vi "MGCC_StaEst_pnjoc.vi"(0 "MeaPha":T2, 1 "Num":T1, 2 "StateVar":dbl[](array[numeric]), 3 "B":dbl[][](array[numeric]), 4 "G":dbl[][](array[numeric])) -> (5 "joc_pn":dbl[][](array[numeric]), 6 "joc_qn":dbl[][](array[numeric]))   [LabVIEW 2016]
uses:
  <vilib>/imath/engines/lvmath2/RunTimeEngine/RunTimeType/NIMS_RunTimeType_From StrictType (excl LVString).vi
  <instcachedir>/0/NIMS_RunTimeType_From StrictType (excl LVString)_BBF44FB49F834B71AF7A14CCEDF8BECD.lvgen/NIMS_RunTimeType_From StrictType (excl LVString)_BBF44FB49F834B71AF7A14CCEDF8BECD_032.vi
  <instcachedir>/0/NIMS_RunTimeType_From StrictType (excl LVString)_BBF44FB49F834B71AF7A14CCEDF8BECD.lvgen/NIMS_RunTimeType_From StrictType (excl LVString)_BBF44FB49F834B71AF7A14CCEDF8BECD_031.vi
  <vilib>/imath/engines/lvmath2/RunTimeEngine/Struct/NIMS_StructSetField.vi
  <instcachedir>/0/NIMS_RunTimeType_From StrictType (excl LVString)_BBF44FB49F834B71AF7A14CCEDF8BECD.lvgen/NIMS_RunTimeType_From StrictType (excl LVString)_BBF44FB49F834B71AF7A14CCEDF8BECD_024.vi
  <vilib>/imath/engines/lvmath2/RunTimeEngine/Struct/NIMS_StructGetField.vi
  <vilib>/imath/engines/lvmath2/RunTimeEngine/RunTimeType/NIMS_RunTimeType_To Numeric.vi
  <instcachedir>/0/NIMS_RunTimeType_To Numeric_19D51BCABB82435A94073491761E42EE.lvgen/NIMS_RunTimeType_To Numeric_19D51BCABB82435A94073491761E42EE_010.vi
  <vilib>/imath/engines/lvmath2/RunTimeEngine/BuiltInFunctions/size/NIMS_I32=size(GM,I32).vi
  <instcachedir>/0/NIMS_I32=size(GM,I32)_122058B1B3294FAEA5DC209B92B394E4.lvgen/NIMS_I32=size(GM,I32)_122058B1B3294FAEA5DC209B92B394E4_005.vi
  <vilib>/imathl/engines/lvmath/Functions/Error Handling/Create Error.vi
  <instcachedir>/0/NIMS_RunTimeType_To Numeric_19D51BCABB82435A94073491761E42EE.lvgen/NIMS_RunTimeType_To Numeric_19D51BCABB82435A94073491761E42EE_008.vi
  <instcachedir>/0/NIMS_RunTimeType_To Numeric_19D51BCABB82435A94073491761E42EE.lvgen/NIMS_RunTimeType_To Numeric_19D51BCABB82435A94073491761E42EE_009.vi
  <vilib>/imath/engines/lvmath2/RunTimeEngine/BuiltInFunctions/zeros/NIMS_M=zeros(I32,I32).vi
  <vilib>/imath/engines/lvmath2/RunTimeEngine/BuiltInFunctions/zeros/NIMS_V=zeros(I32,I32).vi
  <vilib>/imath/engines/lvmath2/RunTimeEngine/RangeToken/NIMS_Range_R2 - Integer.vi
  <instcachedir>/0/NIMS_Range_R2 - Integer_89B873E74E6E489885E44F751DD9C6BF.lvgen/NIMS_Range_R2 - Integer_89B873E74E6E489885E44F751DD9C6BF_000.vi
  <vilib>/imath/engines/lvmath2/RunTimeEngine/CommandStatement/MC_CommandStatement_break.vi
  <vilib>/imath/engines/lvmath2/RunTimeEngine/IndexRead/NIMS M(S,S).vi
  <instcachedir>/0/NIMS M(S,S)_AC51E74150A542F7991B9634C66F3096.lvgen/NIMS M(S,S)_AC51E74150A542F7991B9634C66F3096_002.vi
  <vilib>/imath/engines/lvmath2/RunTimeEngine/RangeToken/NIMS_Range_R2 - Float.vi
  <instcachedir>/0/NIMS_Range_R2 - Float_590A1087448447AEB7F770FC082D3801.lvgen/NIMS_Range_R2 - Float_590A1087448447AEB7F770FC082D3801_000.vi
  <vilib>/imath/engines/lvmath2/RunTimeSupport/NIMS_Error if Not Equal.vi
  <instcachedir>/0/NIMS_Error if Not Equal_43252A79AD05436189442EC0C5E5AB8A.lvgen/NIMS_Error if Not Equal_43252A79AD05436189442EC0C5E5AB8A_000.vi
  <vilib>/imath/engines/lvmath2/RunTimeEngine/IndexRead/NIMS V(S).vi
  <instcachedir>/0/NIMS V(S)_0488751826AF41519A22953C041130DC.lvgen/NIMS V(S)_0488751826AF41519A22953C041130DC_000.vi
  <vilib>/imath/engines/lvmath2/RunTimeEngine/ErrorHandling/NIMS_Create Error From Enums.vi
  <instcachedir>/0/NIMS M(S,S)_AC51E74150A542F7991B9634C66F3096.lvgen/NIMS M(S,S)_AC51E74150A542F7991B9634C66F3096_000.vi
  <vilib>/imath/engines/lvmath2/RunTimeEngine/IndexReplace/NIMS M(S,S)=S.vi
  <instcachedir>/0/NIMS M(S,S)=S_98E40400474E4398B113AE20298B4F82.lvgen/NIMS M(S,S)=S_98E40400474E4398B113AE20298B4F82_000.vi
  <vilib>/imath/engines/lvmath2/RunTimeEngine/IndexReplace/NIMS V(S)=S.vi
  <instcachedir>/0/NIMS V(S)=S_57E16554CB8B4B90AAB163894F717546.lvgen/NIMS V(S)=S_57E16554CB8B4B90AAB163894F717546_000.vi
  <vilib>/imath/engines/lvmath2/RunTimeEngine/NodeEndStatement/NIMS_NodeEndStatement_Output.vi
  <instcachedir>/0/NIMS_NodeEndStatement_Output_53EC0D466D134D7ABD903AC30B43404B.lvgen/NIMS_NodeEndStatement_Output_53EC0D466D134D7ABD903AC30B43404B_002.vi
  <vilib>/imath/engines/lvmath2/RunTimeEngine/ErrorHandling/NIMS_Finalize Error.vi
panel:
  out "error out":errorcluster
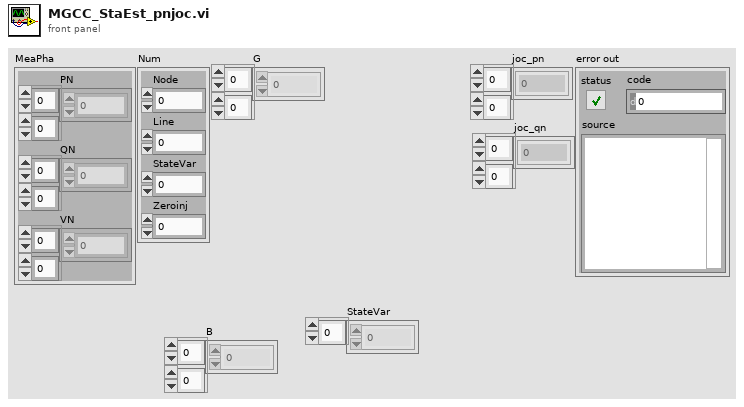
[diagram p1: front panel]
types:
  T1 = cluster{"Node":dbl, "Line":dbl, "StateVar":i32, "Zeroinj":i32}
  T2 = cluster{"PN":i32[][], "QN":i32[][], "VN":i32[][]}
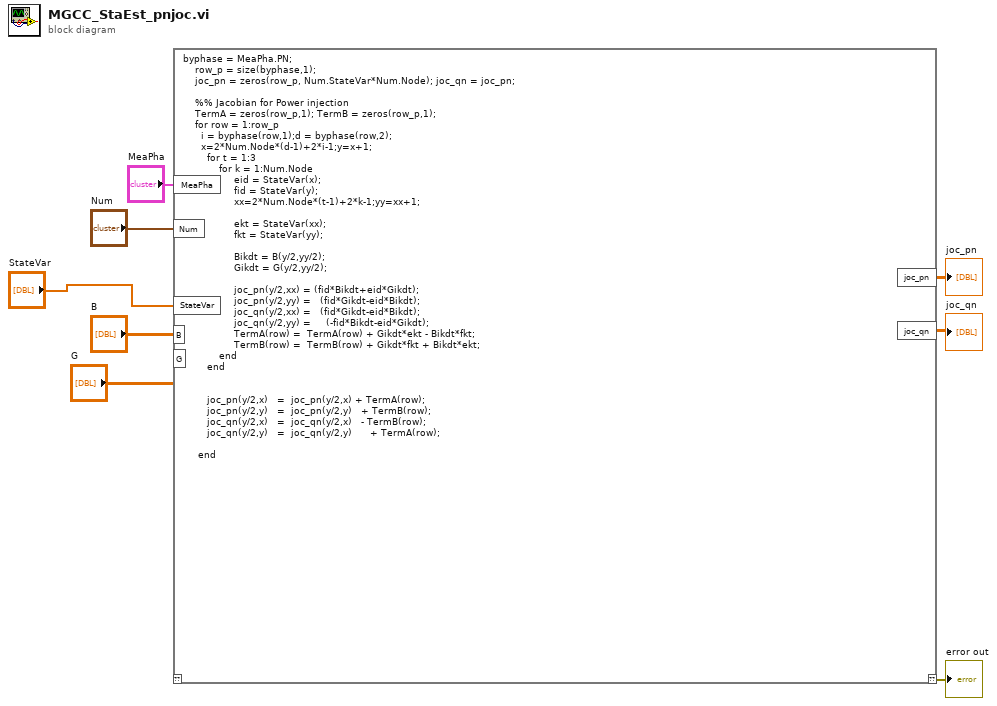
[diagram p0: block diagram]
diagram:
  n1 = mathscript code="byphase = MeaPha.PN;    \n    row_p = size(byphase,1);\n    joc_pn = zeros(row_p, Num.StateVar*Num.Node); joc_qn = joc_pn;\n    \n    %% Jacobian for Power injection\n    TermA = zeros(row_p,1); TermB = zeros(row_p,1);\n    for row = 1:row_p\n      i = byphase(row,1);d = byphase(row,2);\n      x=2*Num.Node*(d-1)+2*i-1;y=x+1;\n        for t = 1:3\n            for k = 1:Num.Node \n                 eid = StateVar(x);\n                 fid = StateVar(y);\n                 xx=2*Num.Node*(t-1)+2*k-1;yy=xx+1;\n\n                 ekt = StateVar(xx);\n                 fkt = StateVar(yy);\n\n                 Bikdt = B(y/2,yy/2);\n                 Gikdt = G(y/2,yy/2);                     \n\n                 joc_pn(y/2,xx) = (fid*Bikdt+eid*Gikdt);  \n                 joc_pn(y/2,yy) =   (fid*Gikdt-eid*Bikdt);  \n                 joc_qn(y/2,xx) =   (fid*Gikdt-eid*Bikdt);  \n                 joc_qn(y/2,yy) =     (-fid*Bikdt-eid*Gikdt); \n                 TermA(row) =  TermA(row) + Gikdt*ekt - Bikdt*fkt;\n                 TermB(row) =  TermB(row) + Gikdt*fkt + Bikdt*ekt;     \n            end\n        end\n        \n        \n        joc_pn(y/2,x)   =  joc_pn(y/2,x) + TermA(row); \n        joc_pn(y/2,y)   =  joc_pn(y/2,y)   + TermB(row);  \n        joc_qn(y/2,x)   =  joc_qn(y/2,x)   - TermB(row);   \n        joc_qn(y/2,y)   =  joc_qn(y/2,y)      + TermA(row);    \n\n     end"("MeaPha"="MeaPha", "Num"="Num", "StateVar"="StateVar", "B"="B", "G"="G") -> ("??"=→"error out":errorcluster, "joc_pn"=→"joc_pn":dbl[][], "joc_qn"=→"joc_qn":dbl[][])  [unwired: 1 in]
